vi "CreateUINetworkStreamRder.vi"(8 "error in (no error)":errorcluster, 11 "IPAddress":string) -> (0 "error out":errorcluster, 3 "Refnum out":refnum<k21>)   [LabVIEW 2018]
uses:
  Controls/Enums/IndicatorsEnum.ctl
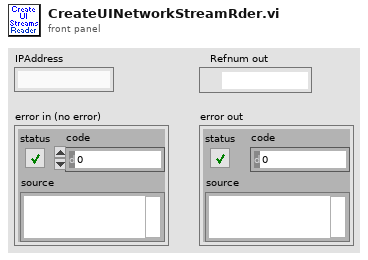
[diagram p1: front panel]
types:
  T1 = typedef "IndicatorsEnum.ctl" = enum16{"NewData", "Px", "Temp", "Power", "Current", "Pelt", "Press", "Supply", "Dials", "HeatCool", "Borders", "MaxTemp", "AllCores", "Paths", "TempVsTime", "UserConfig", "UserConfig2", "CycleCount", "RT_Err", "Stop"}
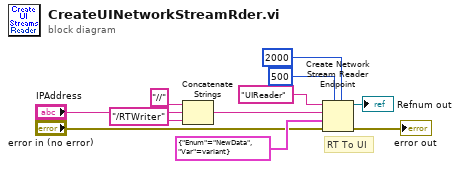
[diagram p0: block diagram]
diagram:
  # "RT To UI"
  n1 = Concatenate Strings("//" ("string"), "IPAddress", "/RTWriter" ("string")) -> (w5:string)
  n2 = Create Network Stream Reader Endpoint(5:2000 ("writer buffer size"), 7:500 ("writer buffer size"), 8:"error in (no error)", 9:cluster{"Enum":T1, "Var":variant} {"Enum"=enum."NewData", "Var"=variant}, 10:w5, 11:"UIReader" ("reader name")) -> (0:→"error out":errorcluster, 3:→"Refnum out":refnum<k21>)  [unwired: 1 in]
